vi "rgr.vi"() -> ()   [LabVIEW 2014]
uses:
  rgr_global.vi
  <vilib>/Instr/_visa.llb/VISA Configure Serial Port (Instr).vi
  <vilib>/Analysis/NI_AAL_SigProc.lvlib
panel:
  in  "Tab Control":enum32{"Спектр", "Настройки"}(tab)
  out "Характеристика":cluster{"Y":dbl[], "Y":dbl[]}[](graph)
  out "Накопление":bool
  out "Время накопления, с":dbl
  in  "Время накопления при замере, с.":dbl
  in  "сбрасывать при измерении":bool
  in  "Сброс":bool
  in  "Накопление":bool
  out "Результаты":string[][](table)
  out "Slide":u8(slide) scale=0.0..9.0
  in  "замер":bool
  out "График спектра":dbl[][](graph)
  out "Текущая температура":dbl(slide) scale=-10.0..100.0
  out "Ближайший пик":dbl
  out "Байт прочитано":u32
  in  "Порог пика":dbl=-0.75 format="%0.2f"
  in  "Ширина пика":i32=50 min=3
  out "Байт в порту":u32
  out "Парсер: канал":i32
  out "Парсер: скорость":i32
  out "Последняя посылка":string
  in  "Скорость":u32=115200
  in  "Порт":refnum<visa-resource-name>="COM104"
  out "Последнняя ошибка":errorcluster
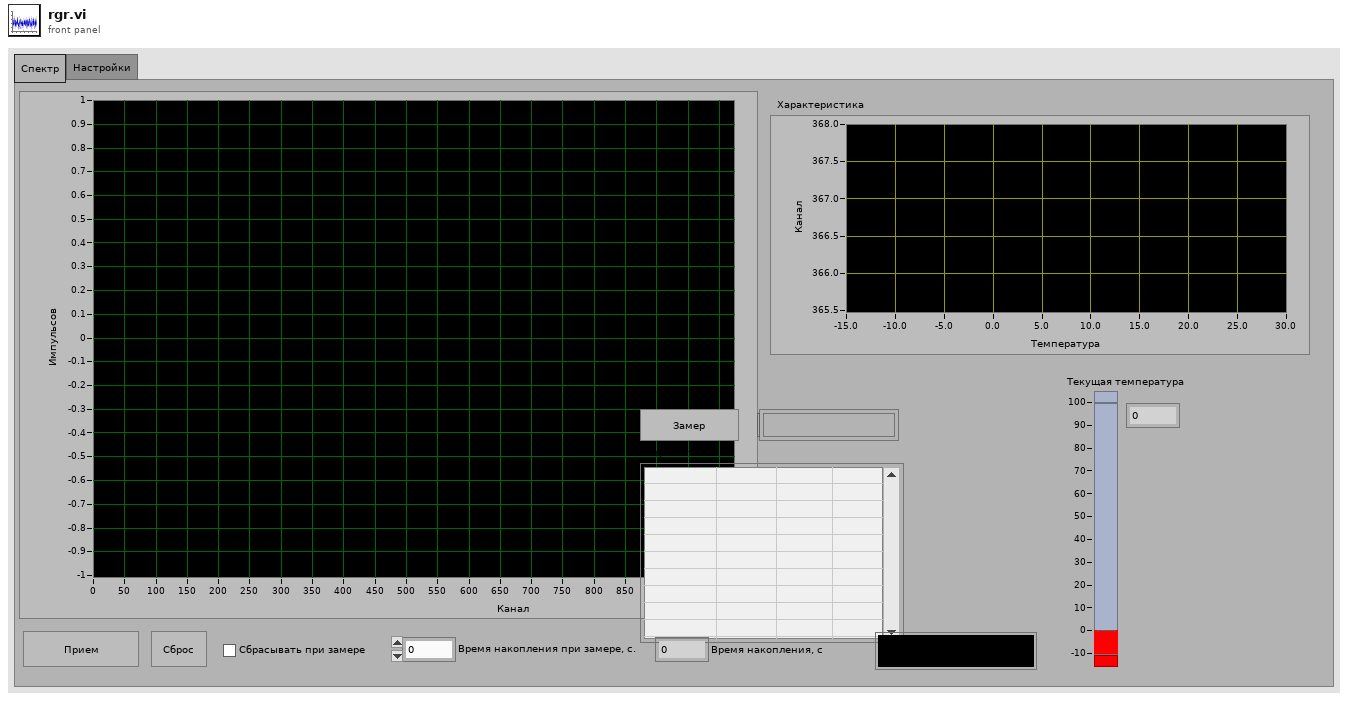
[diagram p1: front panel]
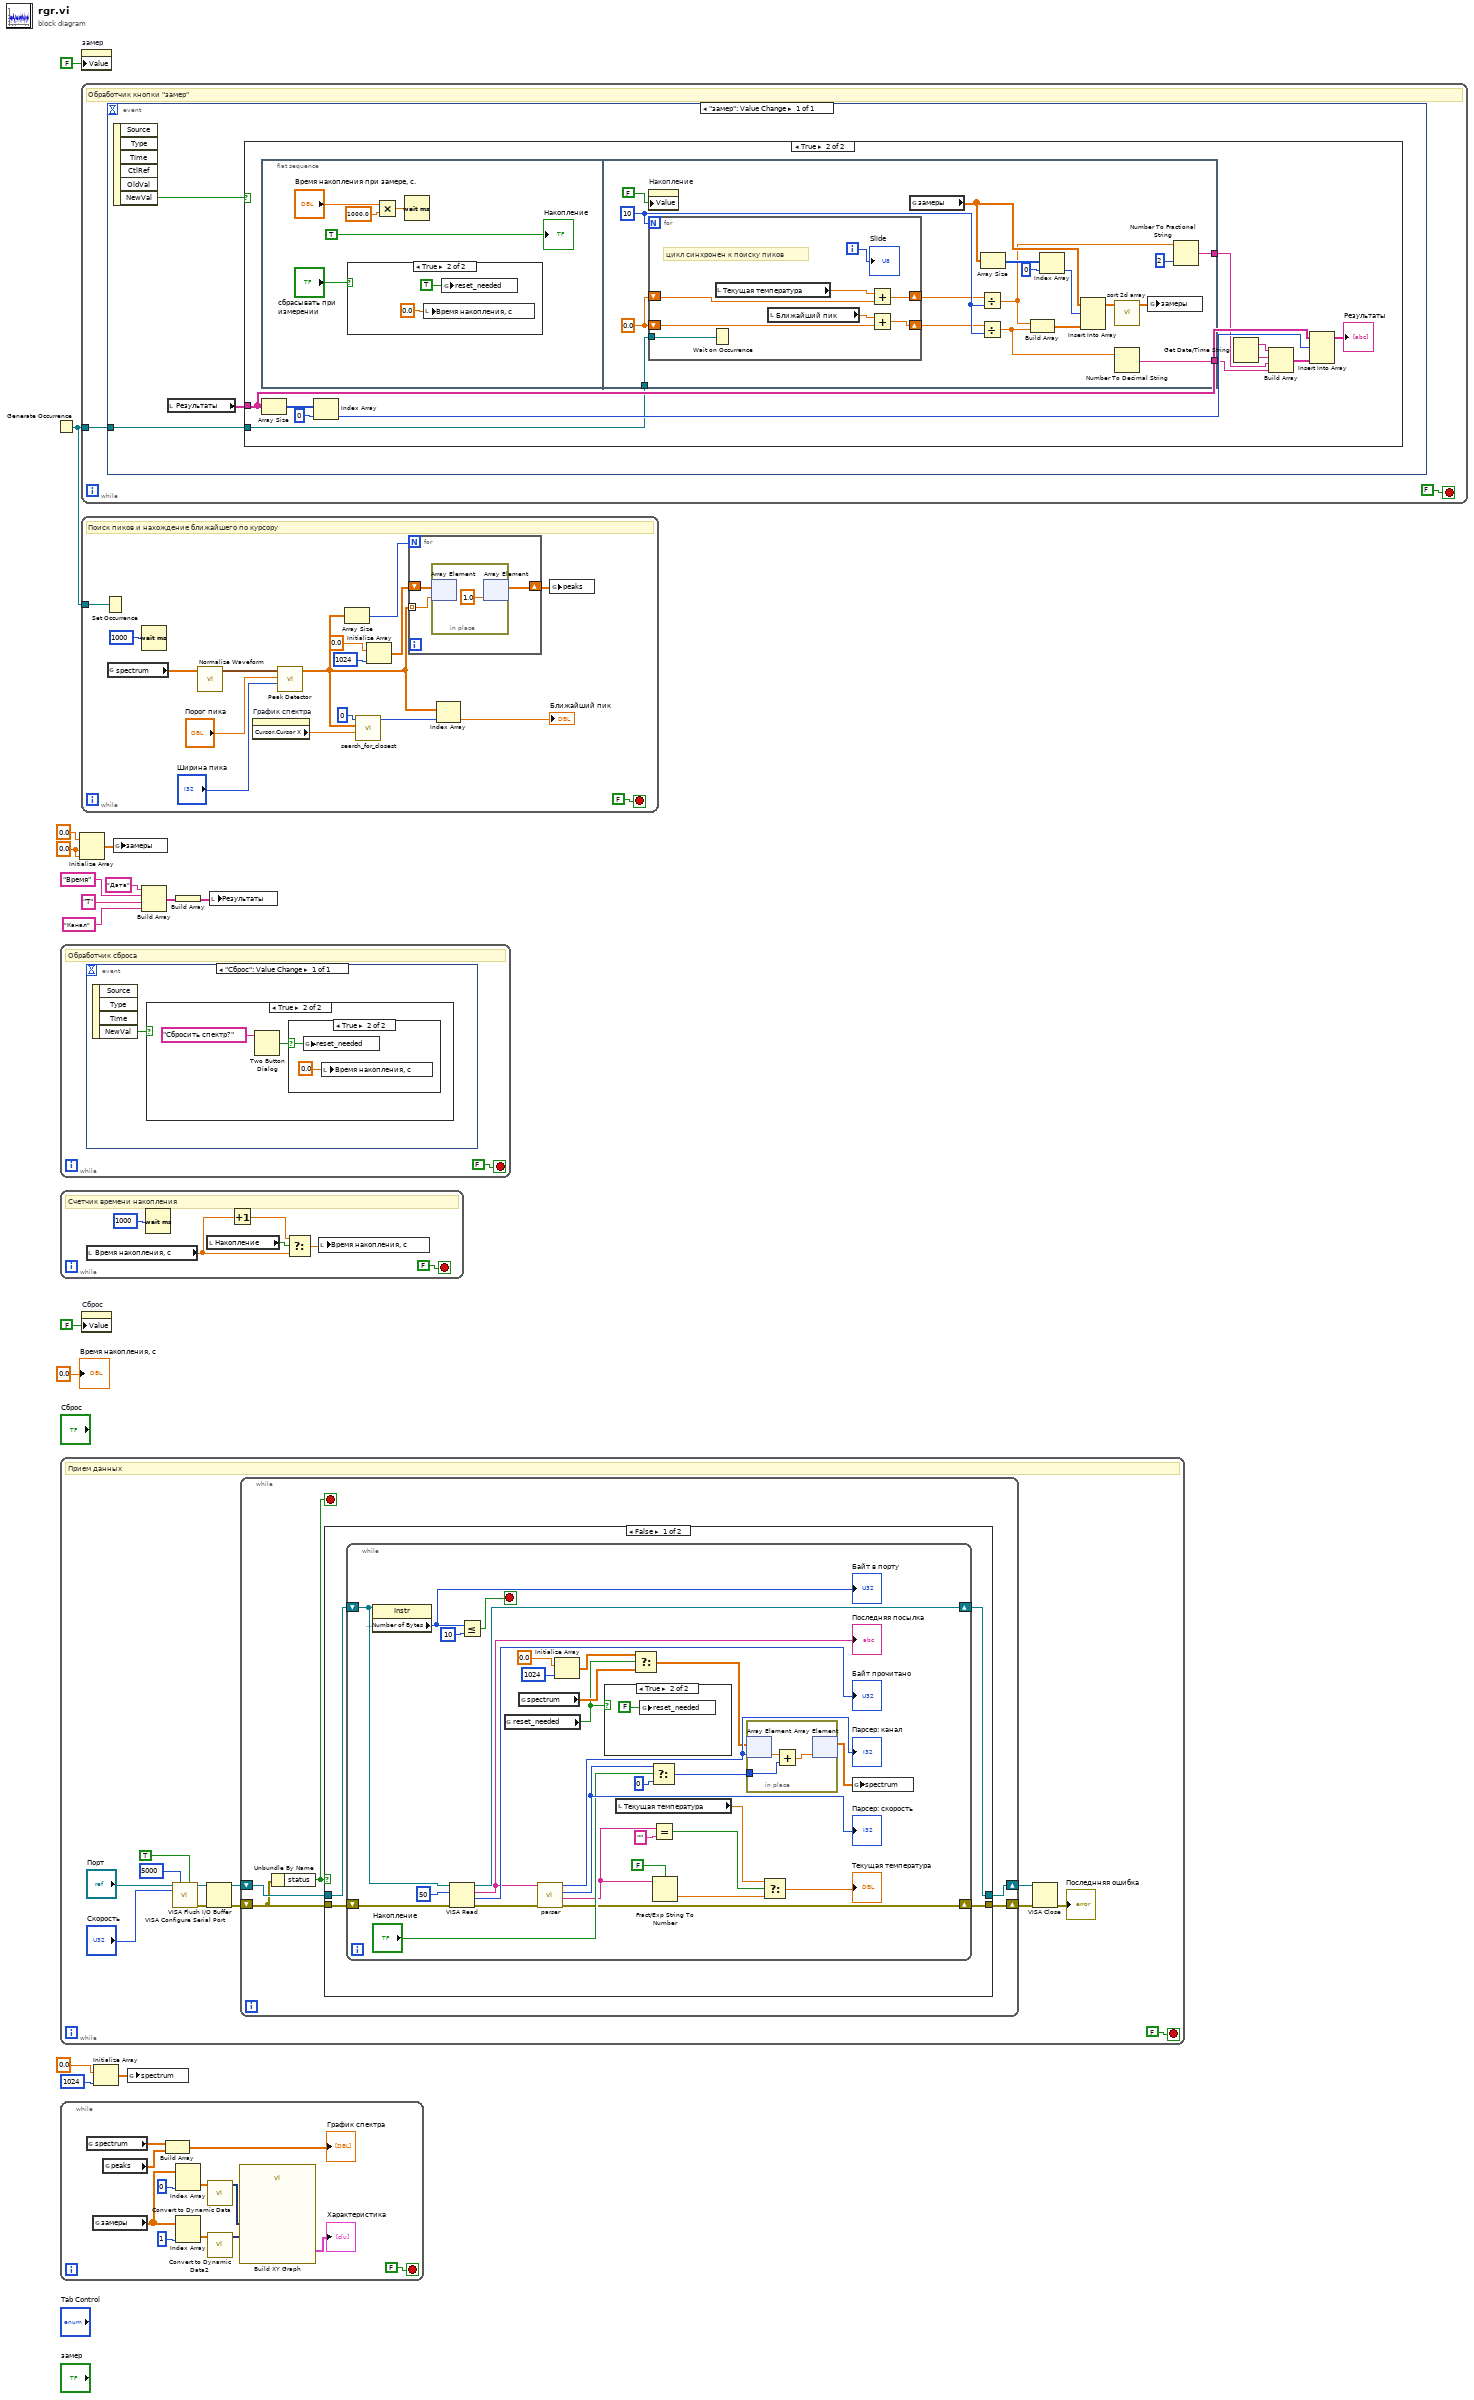
[diagram p0: block diagram]
diagram:
  w2 = 0.0
  n1 = Generate Occurrence() -> (w13:refnum<k4>)
  n2 = while {
    stop <- FALSE stop-if-true
    # "Обработчик сброса"
    n3 = event shown="[0] \"Сброс\": Value Change" {
      selector: _ -> [_]
      dyn-events: _ -> [_]
      timeout: _ -> [_]
      event "Сброс": Value Change {
        n4 = event-data() -> ("NewVal"=w18:bool)  [unwired: 1 in, 3 out]
        n5 = case shown="True" w18 {
          frame False {
          }
          frame True {
            n6 = Two Button Dialog(message="Сбросить спектр?") -> (T button?=w19:bool)  [unwired: 2 in]
            n7 = case shown="True" w19 {
              selector: w19 -> [_ w22]
              frame False {
              }
              frame True {
                n8 = global write "rgr_global.vi" "reset_needed"(w22) -> ()
                n9 = local write "Время накопления, с"(0.0 ("Время накопления, с")) -> ()
              }
            }
          }
        }
      }
    }
  }
  n10 = while {
    stop <- FALSE stop-if-true
    # "Счетчик времени накопления"
    n11 = local read "Время накопления, с"() -> (w23:dbl)
    n12 = Wait (ms)(milliseconds to wait=u32 1000) -> ()  [unwired: 1 out]
    n13 = local read "Накопление"() -> (w26:bool)
    n14 = Increment(x=w23) -> (x+1=w24:dbl)
    n15 = Select(t=w24, s=w26, f=w23) -> (s? t:f=w25:dbl)
    n16 = local write "Время накопления, с"(w25) -> ()
  }
  n17 = while {
    stop <- FALSE stop-if-true
    # "Прием данных"
    n18 = call-poly "VISA Configure Serial Port"("VISA resource name"="Порт", "timeout (10sec)"=u32 5000, "Enable Termination\nChar (T)"=TRUE ("Enable Termination\nChar (T)"), "baud rate (9600)"="Скорость") -> ("VISA resource name out"=w32:refnum<visa-resource-name>, "error out"=w30:errorcluster)  [unwired: 10 in]
    n19 = VISA Flush I/O Buffer(VISA resource name=w32, error in (no error)=w30) -> (VISA resource name out=w31:refnum<visa-resource-name>, error out=w29:errorcluster)  [unwired: 1 in]
    n20 = while {
      shift-right: [w45] -> w37
      shift-left: w31 -> [w44]
      shift-right: [w43] -> w36
      shift-left: w29 -> [w42]
      stop <- w41 stop-if-true
      n21 = Unbundle By Name(w42) -> ("status"=w41:bool)
      n22 = case shown="False" w41 {
        tunnel: [w47 w84] -> w45
        tunnel: w42 -> [w49 w85]
        tunnel: w44 -> [w46 w84]
        tunnel: [w48 w85] -> w43
        frame False {
          n23 = while {
            shift-right: [w57] -> w48
            shift-left: w49 -> [w79]
            shift-right: [w77] -> w47
            shift-left: w46 -> [w71]
            stop <- w72 stop-if-true
            n24 = property class="Instr"(reference=w71) -> ("Serial Settings:Number of Bytes at Serial Port"=w74:u32)  [unwired: 1 in, 2 out]
            "Байт в порту" <- w74
            n25 = VISA Read(VISA resource name=w71, byte count=u32 50, error in (no error)=w79) -> (VISA resource name out=w77:refnum<visa-resource-name>, read buffer=w59:string, return count=→"Байт прочитано":u32, error out=w58:errorcluster)
            "Последняя посылка" <- w59
            n26 = Less Or Equal?(x=w74, y=u32 10) -> (x <= y?=w72:bool)
            n27 = global read "rgr_global.vi" "reset_needed"() -> (w60:bool)
            n28 = global read "rgr_global.vi" "spectrum"() -> (w62:dbl[])
            n29 = call "parser.vi"("error in"=w58, "входная посылка"=w59) -> ("error out"=w57:errorcluster, "температура"=w52:string, "Парсер: скорость"=w70:i32, "Парсер: канал"=w78:i32)  [unwired: 6 in]
            "Парсер: канал" <- w78
            "Парсер: скорость" <- w70
            n30 = Initialize Array(0.0 ("element"), 1024 ("dimension size")) -> (w64:dbl[])
            n31 = case shown="True" w60 {
              frame False {
              }
              frame True {
                n32 = global write "rgr_global.vi" "reset_needed"(FALSE ("reset_needed")) -> ()
              }
            }
            n33 = local read "Текущая температура"() -> (w54:dbl)
            n34 = Select(t=w64, s=w60, f=w62) -> (s? t:f=w63:dbl[])
            n35 = Select(t=w70, s="Накопление", f=0) -> (s? t:f=w68:i32)
            n36 = Equal?(x=w52, y="") -> (x = y?=w55:bool)
            n37 = Fract/Exp String To Number(use system decimal point (T)=FALSE, string=w52) -> (number=w51:dbl)  [unwired: 2 in, 1 out]
            n38 = in-place {
              in-place-border: w68 -> [w82]
              n39 = in-place-array #1(w63, w78) -> (w83:dbl)
              n40 = Add(x=w83, y=w82) -> (x+y=w81:dbl)
              n41 = in-place-array #1(w81) -> (w61:dbl[])  [unwired: 1 out]
            }
            n42 = Select(t=w54, s=w55, f=w51) -> (s? t:f=→"Текущая температура":dbl)
            n43 = global write "rgr_global.vi" "spectrum"(w61) -> ()
          }
        }
        frame True {
        }
      }
    }
    n44 = VISA Close(VISA resource name=w37, error in (no error)=w36) -> (error out=→"Последнняя ошибка":errorcluster)
  }
  n45 = while {
    stop <- FALSE stop-if-true
    n46 = global read "rgr_global.vi" "spectrum"() -> (w95:dbl[])
    n47 = global read "rgr_global.vi" "замеры"() -> (w88:dbl[][])
    n48 = global read "rgr_global.vi" "peaks"() -> (w94:dbl[])
    n49 = Build Array(w95, w94) -> (→"График спектра":dbl[][])
    n50 = Index Array(array=w88, index (col)=0 ("disabled index (col)")) -> (element=w91:dbl[])  [unwired: 1 in]
    n51 = Index Array(array=w88, index (col)=1) -> (element=w87:dbl[])  [unwired: 1 in]
    n52 = call "Convert to Dynamic Data"("Array"=w91) -> ("Dynamic Data Type"=w90:dynamicdata)  [unwired: 3 in]
    n53 = call "Convert to Dynamic Data2"("Array"=w87) -> ("Dynamic Data Type"=w86:dynamicdata)  [unwired: 3 in]
    n54 = call "Build XY Graph"("Y Input"=w86, "X Input"=w90) -> ("XY Graph"=→"Характеристика":cluster{"X":dbl[], "Y":dbl[]}[])  [unwired: 8 in, 1 out]
  }
  n55 = Initialize Array(0.0, w2, w2) -> (w4:dbl[][])
  n56 = property on="замер" class="Bool (strict)"("Value"=FALSE ("замер")) -> ()  [unwired: 2 in, 2 out]
  n57 = while {
    tunnel: w13 -> [w98]
    stop <- FALSE stop-if-true
    # "Обработчик кнопки \"замер\""
    n58 = event shown="[0] \"замер\": Value Change" {
      selector: _ -> [_]
      dyn-events: _ -> [_]
      timeout: _ -> [_]
      tunnel: w98 -> [w101]
      event "замер": Value Change {
        n59 = event-data() -> ("NewVal"=w102:bool)  [unwired: 1 in, 5 out]
        n60 = local read "Результаты"() -> (w100:string[][])
        n61 = case shown="True" w102 {
          tunnel: w101 -> [_ w105]
          tunnel: w100 -> [_ w111]
          frame False {
          }
          frame True {
            n62 = flat-sequence {
              tunnel: [w123] -> w104
              tunnel: w105 -> [w138]
              tunnel: [w130] -> w103
              frame #0 {
                n63 = case shown="True" "сбрасывать при измерении" {
                  frame False {
                  }
                  frame True {
                    n64 = local write "Время накопления, с"(0.0 ("Время накопления, с")) -> ()
                    n65 = global write "rgr_global.vi" "reset_needed"(TRUE ("Сброс")) -> ()
                  }
                }
                n66 = Multiply(x="Время накопления при замере, с.", y=1000.0) -> (x*y=w115:dbl)
                n67 = Wait (ms)(milliseconds to wait=w115) -> ()  [unwired: 1 out]
                "Накопление" <- TRUE ("Накопление")
              }
              frame #1 {
                w128 = 0.0
                w131 = 10
                n68 = property on="Накопление" class="Bool (strict)"("Value"=FALSE ("Накопление")) -> ()  [unwired: 2 in, 2 out]
                n69 = for {
                  N: w131 -> [_]
                  shift-right: [w146] -> w124
                  shift-left: w128 -> [w145]
                  tunnel: w138 -> [w142]
                  shift-right: [w140] -> w125
                  shift-left: w128 -> [w139]
                  i -> [w144]
                  # "цикл синхронен к поиску пиков"
                  n70 = Wait on Occurrence(2:w142) -> ()  [unwired: 2 in, 1 out]
                  n71 = local read "Текущая температура"() -> (w141:dbl)
                  n72 = local read "Ближайший пик"() -> (w143:dbl)
                  n73 = Add(x=w141, y=w139) -> (x+y=w140:dbl)
                  n74 = Add(x=w143, y=w145) -> (x+y=w146:dbl)
                  "Slide" <- w144
                }
                n75 = global read "rgr_global.vi" "замеры"() -> (w136:dbl[][])
                n76 = Divide(x=w125, y=w131) -> (x/y=w122:dbl)
                n77 = Divide(x=w124, y=w131) -> (x/y=w129:dbl)
                n78 = Array Size(array=w136) -> (size(s)=w134:i32[])
                n79 = Build Array(w122, w129) -> (w135:dbl[])
                n80 = Index Array(array=w134, index=0) -> (element=w132:i32)
                n81 = Insert Into Array(array=w136, index (row)=w132, new element=w135) -> (w127:dbl[][])  [unwired: 1 in]
                n82 = call "sort 2d array.vi"("input"=w127) -> ("output"=w126:dbl[][])  [unwired: 10 in]
                n83 = Number To Decimal String(number=w129) -> (decimal integer string=w130:string)  [unwired: 1 in]
                n84 = global write "rgr_global.vi" "замеры"(w126) -> ()
                n85 = Number To Fractional String(number=w122, precision (6)=i16 2) -> (F-format string=w123:string)  [unwired: 2 in]
              }
            }
            n86 = Array Size(array=w111) -> (size(s)=w113:i32[])
            n87 = Index Array(array=w113, index=0) -> (element=w108:i32)
            n88 = Get Date/Time String() -> (date string=w107:string, time string=w106:string)  [unwired: 3 in]
            n89 = Build Array(w107, w106, w104, w103) -> (w110:string[])
            n90 = Insert Into Array(array=w111, index (row)=w108, new element=w110) -> (→"Результаты":string[][])  [unwired: 1 in]
          }
        }
      }
    }
  }
  n91 = while {
    tunnel: w13 -> [w150]
    stop <- FALSE stop-if-true
    # "Поиск пиков и нахождение ближайшего по курсору"
    n92 = Set Occurrence(w150) -> ()
    n93 = global read "rgr_global.vi" "spectrum"() -> (w149:dbl[])
    n94 = Wait (ms)(milliseconds to wait=u32 1000) -> ()  [unwired: 1 out]
    n95 = call <vilib>:"Normalize Waveform.vi"("waveform in"=w149) -> ("normalized waveform"=w161:waveform(dbl))  [unwired: 7 in, 3 out]
    n96 = property on="График спектра" class="WFGraph (strict)"() -> ("Cursor.Cursor X"=w153:dbl)  [unwired: 2 in, 2 out]
    n97 = call <vilib>:"Peak Detector.vi"("width"="Ширина пика", "threshold"="Порог пика", "X"=w161) -> ("Locations"=w154:dbl[])  [unwired: 4 in, 4 out]
    n98 = Array Size(array=w154) -> (size(s)=w156:i32)
    n99 = call "search_for_closest.vi"("search center"=w153, "input array"=w154, "start index"=0 ("index")) -> ("closest element"=w152:i32)  [unwired: 8 in]
    n100 = Initialize Array(0.0 ("element"), 1024 ("dimension size")) -> (w157:dbl[])
    n101 = for {
      N: w156 -> [_]
      tunnel: w154 -> [w165] mode=indexing
      shift-right: [w164] -> w148
      shift-left: w157 -> [w166]
      n102 = in-place {
        n103 = in-place-array #2(w166, w165) -> ()  [unwired: 1 out]
        n104 = in-place-array #2(1.0 ("element")) -> (w164:dbl[])  [unwired: 1 out]
      }
    }
    n105 = Index Array(array=w154, index=w152) -> (element=→"Ближайший пик":dbl)
    n106 = global write "rgr_global.vi" "peaks"(w148) -> ()
  }
  n107 = property on="Сброс" class="Bool (strict)"("Value"=FALSE ("Сброс")) -> ()  [unwired: 2 in, 2 out]
  n108 = Initialize Array(0.0 ("element"), 1024 ("dimension size")) -> (w6:dbl[])
  n109 = global write "rgr_global.vi" "замеры"(w4) -> ()
  n110 = global write "rgr_global.vi" "spectrum"(w6) -> ()
  n111 = Build Array("Дата", "Время", "T", "Канал") -> (w12:string[])
  n112 = Build Array(w12) -> (w7:string[][])
  n113 = local write "Результаты"(w7) -> ()
  "Время накопления, с" <- 0.0 ("Время накопления, с")
